vi "Run.vi"(7 "Team Index":i32, 8 "Column":i32, 9 "Row":i32, 10 "View":i32[](array[numeric]) caption="View (Team Index, -1: empty)", 11 "Test In":refnum<class "Pattern 5.lvclass">) -> (0 "Replicated":refnum<class "Square.lvclass">, 1 "Direction":T1, 2 "Action":T2, 3 "Test Out":refnum<class "Pattern 5.lvclass">)   [LabVIEW 2015, in "Pattern 5.lvclass"]
uses:
  Pattern 5.lvclass
  Type Defs/Action Enum.ctl
  Type Defs/Direction Enum.ctl
  Square/Square.lvclass
  Pattern 5.lvclass/Pattern 5.ctl
  Type Defs/SB Type Defs.lvlib
  Common/Common.lvlib
panel:
  # "NW\nN\nNE\nE\nSE\nS\nSW\nW"
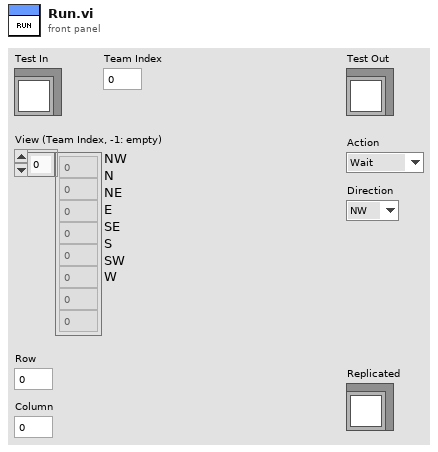
[diagram p1: front panel]
types:
  T1 = typedef "SB Type Defs.lvlib/Direction Enum.ctl" = enum16{"NW", "N", "NE", "E", "SE", "S", "SW", "W"}
  T2 = typedef "SB Type Defs.lvlib/Action Enum.ctl" = enum16{"Wait", "Move", "Attack", "Replicate"}
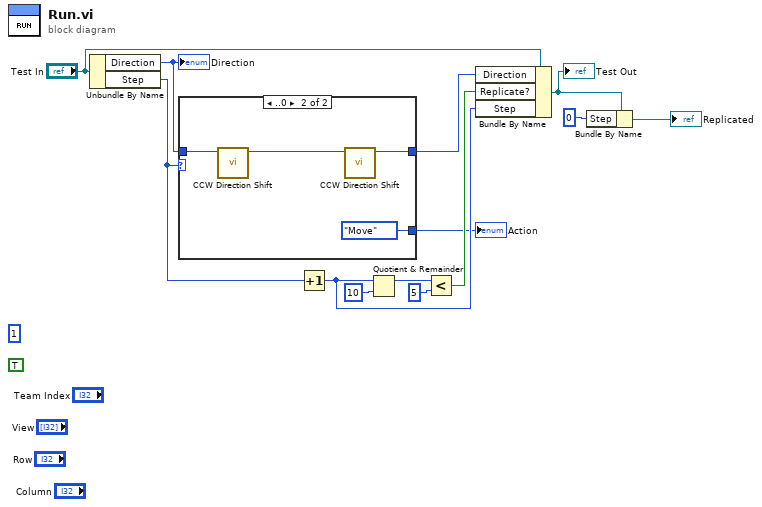
[diagram p0: block diagram]
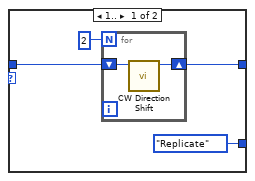
[diagram p2: hidden frame]
diagram:
  (unwired) 1
  (unwired) TRUE ("x < y?")
  n1 = Unbundle By Name("Test In") -> ("Direction"=w2:T1, "Step"=w4:i32)
  "Direction" <- w2
  n2 = case shown="..0" w4 {
    tunnel: [Action_Enum."Replicate" ("Action") Action_Enum."Move" ("f")] -> w3
    tunnel: w2 -> [w15 w22]
    tunnel: [w14 w21] -> w1
    frame 1.. {
      n3 = for {
        N: 2 -> [_]
        shift-right: [w19] -> w14
        shift-left: w15 -> [w18]
        n4 = call "CW Direction Shift.vi"("Direction"=w18) -> ("Numeric"=w19:i32)  [unwired: 10 in]
      }
    }
    frame ..0 {
      n5 = call "CCW Direction Shift.vi"("Direction"=w22) -> ("Numeric"=w20:i32)  [unwired: 10 in]
      n6 = call "CCW Direction Shift.vi"("Direction"=w20) -> ("Numeric"=w21:i32)  [unwired: 10 in]
    }
  }
  "Action" <- w3
  n7 = Increment(x=w4) -> (x+1=w7:i32)
  n8 = Quotient & Remainder(x=w7, y=10) -> (x-y*floor(x/y)=w9:i32)  [unwired: 1 out]
  n9 = Less?(x=w9, y=5) -> (x < y?=w5:bool)
  n10 = Bundle By Name(cluster="Test In", "Direction"=w1, "Replicate?"=w5, "Step"=w7) -> (w12:refnum<class "Pattern 5.lvclass">)
  "Test Out" <- w12
  n11 = Bundle By Name(cluster=w12, "Step"=0) -> (→"Replicated":refnum<class "Pattern 5.lvclass">)
